vi "Dashboard Main.vi"() -> ()   [LabVIEW 2015]
uses:
  <vilib>/Utility/miscctls.llb/LVRowAndColumnTypeDef.ctl
  <vilib>/event_ctls.llb/eventvkey.ctl
  <vilib>/Rock Robotics/WPI/Dashboard/WPI_DashboardLogging Global.vi
  <vilib>/Rock Robotics/Network Tables/NT Read Numeric Array.vi
  <vilib>/Utility/config.llb/Write Key (String).vi
  <vilib>/Utility/config.llb/Write Key (I32).vi
  <vilib>/Utility/config.llb/NI_LVConfig.lvlib
panel:
  out "Robot IP":string
  in  "stop":bool
  in  "TCP":refnum<k5>
  out "Camera IP":string
  out "Image Message":string="Timeout in Camera Communications"
  in  "Dashboard Tab":T1(tab)
  in  "Select Auto":string(combo)
  out "NT Connection":bool
  in  "Camera Settings":T2={"Frame Rate"=30, "Compression"=30, "Size"=1} {"Frame Rate" scale=1.0..30.0; "Size" items=["640x480", "320x240", "160x120"]}
  out "MotorChart R":cluster{"Numeric":dbl, "Numeric":dbl}(graph)
  out "MotorChart L":T3(graph)
  out "MotorSliders R":cluster{"MotorSlide1":dbl, "MotorSlide2":dbl} {"MotorSlide2" scale=-1.0..1.0 scale format="%#_2e"; "MotorSlide1" scale=-1.0..1.0 scale format="%#_2e"}
  out "MotorSliders L":T4 {"MotorSlide4 2" scale=0.0..14.0 scale format="%#_2e"; "MotorSlide2" scale=-1.0..1.0 scale format="%#_2e"; "MotorSlide1" scale=-1.0..1.0 scale format="%#_2e"}
  out "Gyro":dbl(knob) scale=0.0..360.0
  out "JS1 Z":dbl(slide) scale=-1.0..1.0 scale format="%#_2e"
  out "JS1 Graph":cluster{"X":dbl, "Y":dbl}[](graph)
  out "JS1 Buttons":T5
  out "JS2 Z":dbl(slide) scale=-1.0..1.0 scale format="%#_2e"
  out "JS2 Graph":cluster{"X":dbl, "Y":dbl}[](graph)
  out "JS2 Buttons":T5
  out "Mode":T6(ring)=enum."Auto Disabled"
  in  "DB Camera Config":bool
  out "fps":dbl format="%#.1g"
  out "Mbps":dbl format="%#.1g"
  out "Mbps LED":bool
  in  "Vision":u16(ring) items=["Camera Off", "USB Camera SW", "USB Camera HW", "IP Camera"]
  in  "Rec Mode":enum32{"Stop", "Record", "Playback"}(radio)
  out "Camera Image":T7(plugin-control)
  out "Background":bool
  in  "DB/String 9":string
  in  "DB/String 8":string
  in  "DB/String 7":string
  in  "DB/String 6":string
  in  "DB/String 5":string
  in  "DB/String 4":string
  in  "DB/String 3":string
  in  "DB/String 2":string
  in  "DB/String 1":string
  in  "DB/String 0":string
  in  "DB/Slider 0":dbl(slide) scale=0.0..5.0
  in  "DB/Slider 1":dbl(slide) scale=0.0..5.0
  in  "DB/Slider 2":dbl(slide) scale=0.0..5.0
  in  "DB/Slider 3":dbl(slide) scale=0.0..5.0
  out "DB/LED 3":bool
  out "DB/LED 2":bool
  out "DB/LED 1":bool
  out "DB/LED 0":bool
  in  "DB/Button 3":bool
  in  "DB/Button 2":bool
  in  "DB/Button 1":bool
  in  "DB/Button 0":bool caption="New Name"
  in  "Test Slider":dbl(slide) scale=0.0..100.0 scale format="%#_3g"
  in  "On/Off":bool caption="Solenoid"
  in  "Test Name":u16(ring) items=["Select the test to run..."]
  in  "Test Tree":string(tree)
  in  "Motor":cluster{"Value":dbl, "Enable":bool} {"Value" scale=-1.0..1.0 scale format="%#_3g"}
  out "Progress":T8 {"Test Progress" scale=0.0..100.0}
  in  "Rev/Fwd":cluster{"Forward":bool, "Reverse":bool}
  in  "Test Ring":u16(ring) items=["Monochrome", "Color"]
  out "Cmd Status":string
  in  "Execute Command":bool
  in  "Command Params":string[][](table)
  in  "Command Selection":i32(listbox)
  in  "CheckList":i32(listbox)
  out "Tree":string(tree)
  out "Sorted Particle Scores":T9(array[cluster]) {"Moment Factor" format="%#_3g"; "Aspect Ratio" format="%#_3g"; "Area to CH" format="%#_3g"; "X" format="%#_3g"; "Y" format="%#_3g"}
  out "Detected Targets":T10(array[cluster]) {"Normalized Rect"."Numeric 5" format="%#_2g"; "Normalized Rect"."Numeric 3" format="%#_2g"; "Normalized Rect"."Numeric 2" format="%#_2g"; "Normalized Rect"."Numeric" format="%#_2g"}
  in  "LED Color":T11={"Hue"={101.77223077407461, 133.17163207204948}, "Sat"={151.78571428571428, 255.0}, "Val"={48.571428571428584, 255.0}} {"Hue" scale=0.0..255.0 scale format="%#_3g"}
  out "Masked":T7(plugin-control)
  in  "Viewing Angle":dbl
  # "Left"
  # "Front"
  # "Right"
  # "Battery"
  # "This tab is a great place for autonomous settings and robot-specific values.\nPlace controls and indicators inside this tab and match name to\nDashboard Variables on robot. You can also delete this comment."
  # "Density Profile"
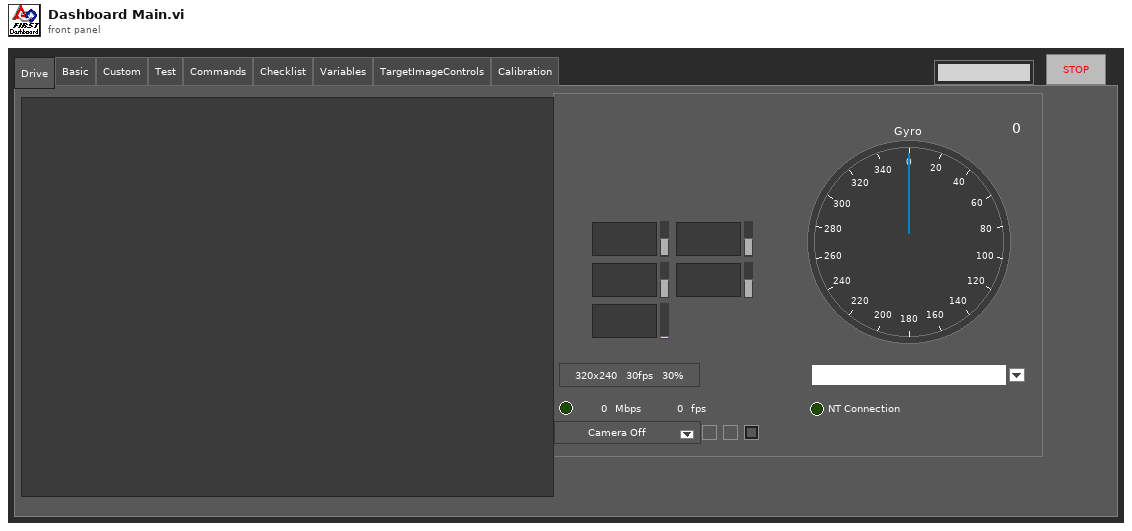
[diagram p1: front panel]
types:
  T1 = enum32{"Drive", "Basic", "Custom", "Test", "Commands", "Checklist", "Variables", "TargetImageControls", "Calibration"}
  T2 = cluster{"Frame Rate":i32, "Compression":i32, "Size":u16}
  T3 = cluster{"Numeric":dbl, "Numeric":dbl, "Battery V":dbl}
  T4 = cluster{"MotorSlide1":dbl, "MotorSlide2":dbl, "MotorSlide4 2":dbl}
  T5 = cluster{bool, bool, bool, bool, bool, bool, bool, bool, bool, bool, bool, bool}
  T6 = enum8{"Tele-Op Disabled", "Tele-Op Enabled", "Auto Disabled", "Auto Enabled", "Test Disabled", "Test Enabled", "Disconnected", "No Code", "E-Stop"}
  T7 = typedef "IMAQ Image.ctl" = refnum<image>
  T8 = cluster{"Test Progress":u8, "Test Progress Text":string}
  T9 = cluster{"Rectangle px":cluster{"Numeric":dbl, "Numeric 2":dbl, "Numeric 3":dbl, "Numeric 5":dbl}, "Aspect Ratio":dbl, "Area to CH":dbl, "X":dbl, "Y":dbl, "Moment Factor":dbl}[]
  T10 = cluster{"Distance (ft)":dbl, "Center":cluster{dbl, dbl}, "Normalized Rect":cluster{"Numeric":dbl, "Numeric 2":dbl, "Numeric 3":dbl, "Numeric 5":dbl}}[]
  T11 = cluster{"Hue":cluster{dbl, dbl}, "Sat":cluster{dbl, dbl}, "Val":cluster{dbl, dbl}}
  T12 = cluster{"IDs":cluster{"RPC field ID":u16, "Unique ID":u16}, "String":string}
  T13 = enum32{"Drive", "Basic", "Custom", "Test", "Commands", "Checklist", "Variables"}
  T14 = enum32{"Drive", "Basic", "Custom", "Test", "Checklist", "Variables"}
  T15 = typedef "Image Type" = u32
  T16 = cluster{"Camera Image":refnum<vi>, "Dashboard Tab":refnum<vi>, "Background":refnum<vi>, "Vision":refnum<vi>, "Rec Mode":refnum<vi>, "Test Slider":refnum<vi>, "On/Off ":refnum<vi>, "Test Ring":refnum<vi>, "Rev/Fwd":refnum<vi>, "Test Name":refnum<vi>, "Motor":refnum<vi>, "Progress":refnum<vi>, "CheckList":refnum<vi>, "Tree":refnum<vi>, "Test Tree":refnum<vi>, "Command Params":refnum<vi>, "Command Selection":refnum<vi>, "Execute Command":refnum<vi>, "Cmd Status":refnum<vi>}
  T17 = cluster{"Error Strings":string, "Disable Counts":cluster{u16, u16}, "Rail Faults":cluster{u16, u16, u16}, "Robot IP":string, "DB Mode":u8, "Event Info":cluster{"Name":string, "Type":u8, "Number":u16, "Replay":u8}, "Camera Addr":string}
  T18 = cluster{"Storage":cluster{"Disk Free":u64, "RAM Block":u32, "RAM free":u32}, "CPU Utilization":cluster{"CPU % ISR":sgl, "CPU % Time Crit":sgl, "CPU % Timed Str":sgl, "CPU % High":sgl, "CPU % Above":sgl, "CPU % Normal":sgl, "CPU % Low":sgl}, "CAN":cluster{"% Bus Utilization":sgl, "Bus Off Cnt":u32, "TX_FIFO Full Cnt":u32, "Receive Error Cnt":u8, "Transmit Error Cnt":u8}, "HID":cluster{"HID Outputs":u32, "Rumble Low":u16, "Rumble High":u16}[]}
  T19 = cluster{"Status bits":cluster{"Test Mode":bool, "Autonomous":bool, "Enabled":bool, "Code Start":bool, "Brownout":bool, "Reserved 2":bool, "Reserved 3":bool, "E-Stop":bool}, "Code Trace":cluster{"Disabled":bool, "TeleOp":bool, "Auto":bool, "Test":bool}, "Controller Type":enum16{"unknown", "cRIO", "roboRio"}, "Code?":enum16{"unknown", "noCode", "code"}, "Battery V":dbl}
  T20 = cluster{"Control Bits":cluster{"TestMode":bool, "Autonomous":bool, "Enabled":bool, "FMS Present":bool, bool, bool, bool, "E-Stop":bool}, "Team Station ":u8, "Countdown":sgl, "Joystick Values":cluster{"Axes":dbl[], "Buttons":bool[], "POVs":i16[]}[]}
  T21 = cluster{"Axes":dbl[], "Buttons":bool[], "POVs":i16[]}[]
  T22 = cluster{"Axes":dbl[], "Buttons":bool[], "POVs":i16[]}
  T23 = cluster{"Buttons[0]":bool, "Buttons[1]":bool, "Buttons[2]":bool, "Buttons[3]":bool, "Buttons[4]":bool, "Buttons[5]":bool, "Buttons[6]":bool, "Buttons[7]":bool, "Buttons[8]":bool, "Buttons[9]":bool, "Buttons[10]":bool, "Buttons[11]":bool}
  T24 = typedef "NI_LVConfig.lvlib/Config Data RefNum.ctl" = refnum<k1>
  T25 = cluster{"Operation":enum16{"Update", "Clear"}, "Color Box":u32}[]
  T26 = typedef "eventvkey.ctl" = enum16{"ASCII", "Enter", "Return", "Shift", "Ctrl", "Alt", "Cmd", "Opt", "Caps", "NumLock", "Clear", "Break", "Up", "Down", "Left", "Right", "Insert", "Delete", "Home", "End", "PageUp", "PageDown", "Escape", "Help", "Pause", "ScrollLock", "F1", "F2", "F3", "F4", "F5", "F6", "F7", "F8", "F9", "F10", "F11", "F12", "F13", "F14", "F15", "F16", "F17", "F18", "F19", "F20", "F21", "F22", "F23", "F24", "Play", "VolumeUp", "VolumeDown", "Mute", "Two Byte Char"}
  T27 = cluster{"Image Size":bool, "Image Type":bool, "Pixel Value":bool, "ROI Information":bool, "Zoom Factor":bool}
  T28 = enum8{"Enabled", "Disabled", "Disabled and Grayed Out"}
  T29 = cluster{"Operation":enum16{"Update", "Clear"}, "Color Box":u32}
  T30 = typedef "LVRowAndColumnTypeDef.ctl" = cluster{"Row":i32, "Column":i32}
  T31 = cluster{"Shift":bool, "Ctrl":bool, "Alt":bool, "Cmd":bool, "Opt":bool}
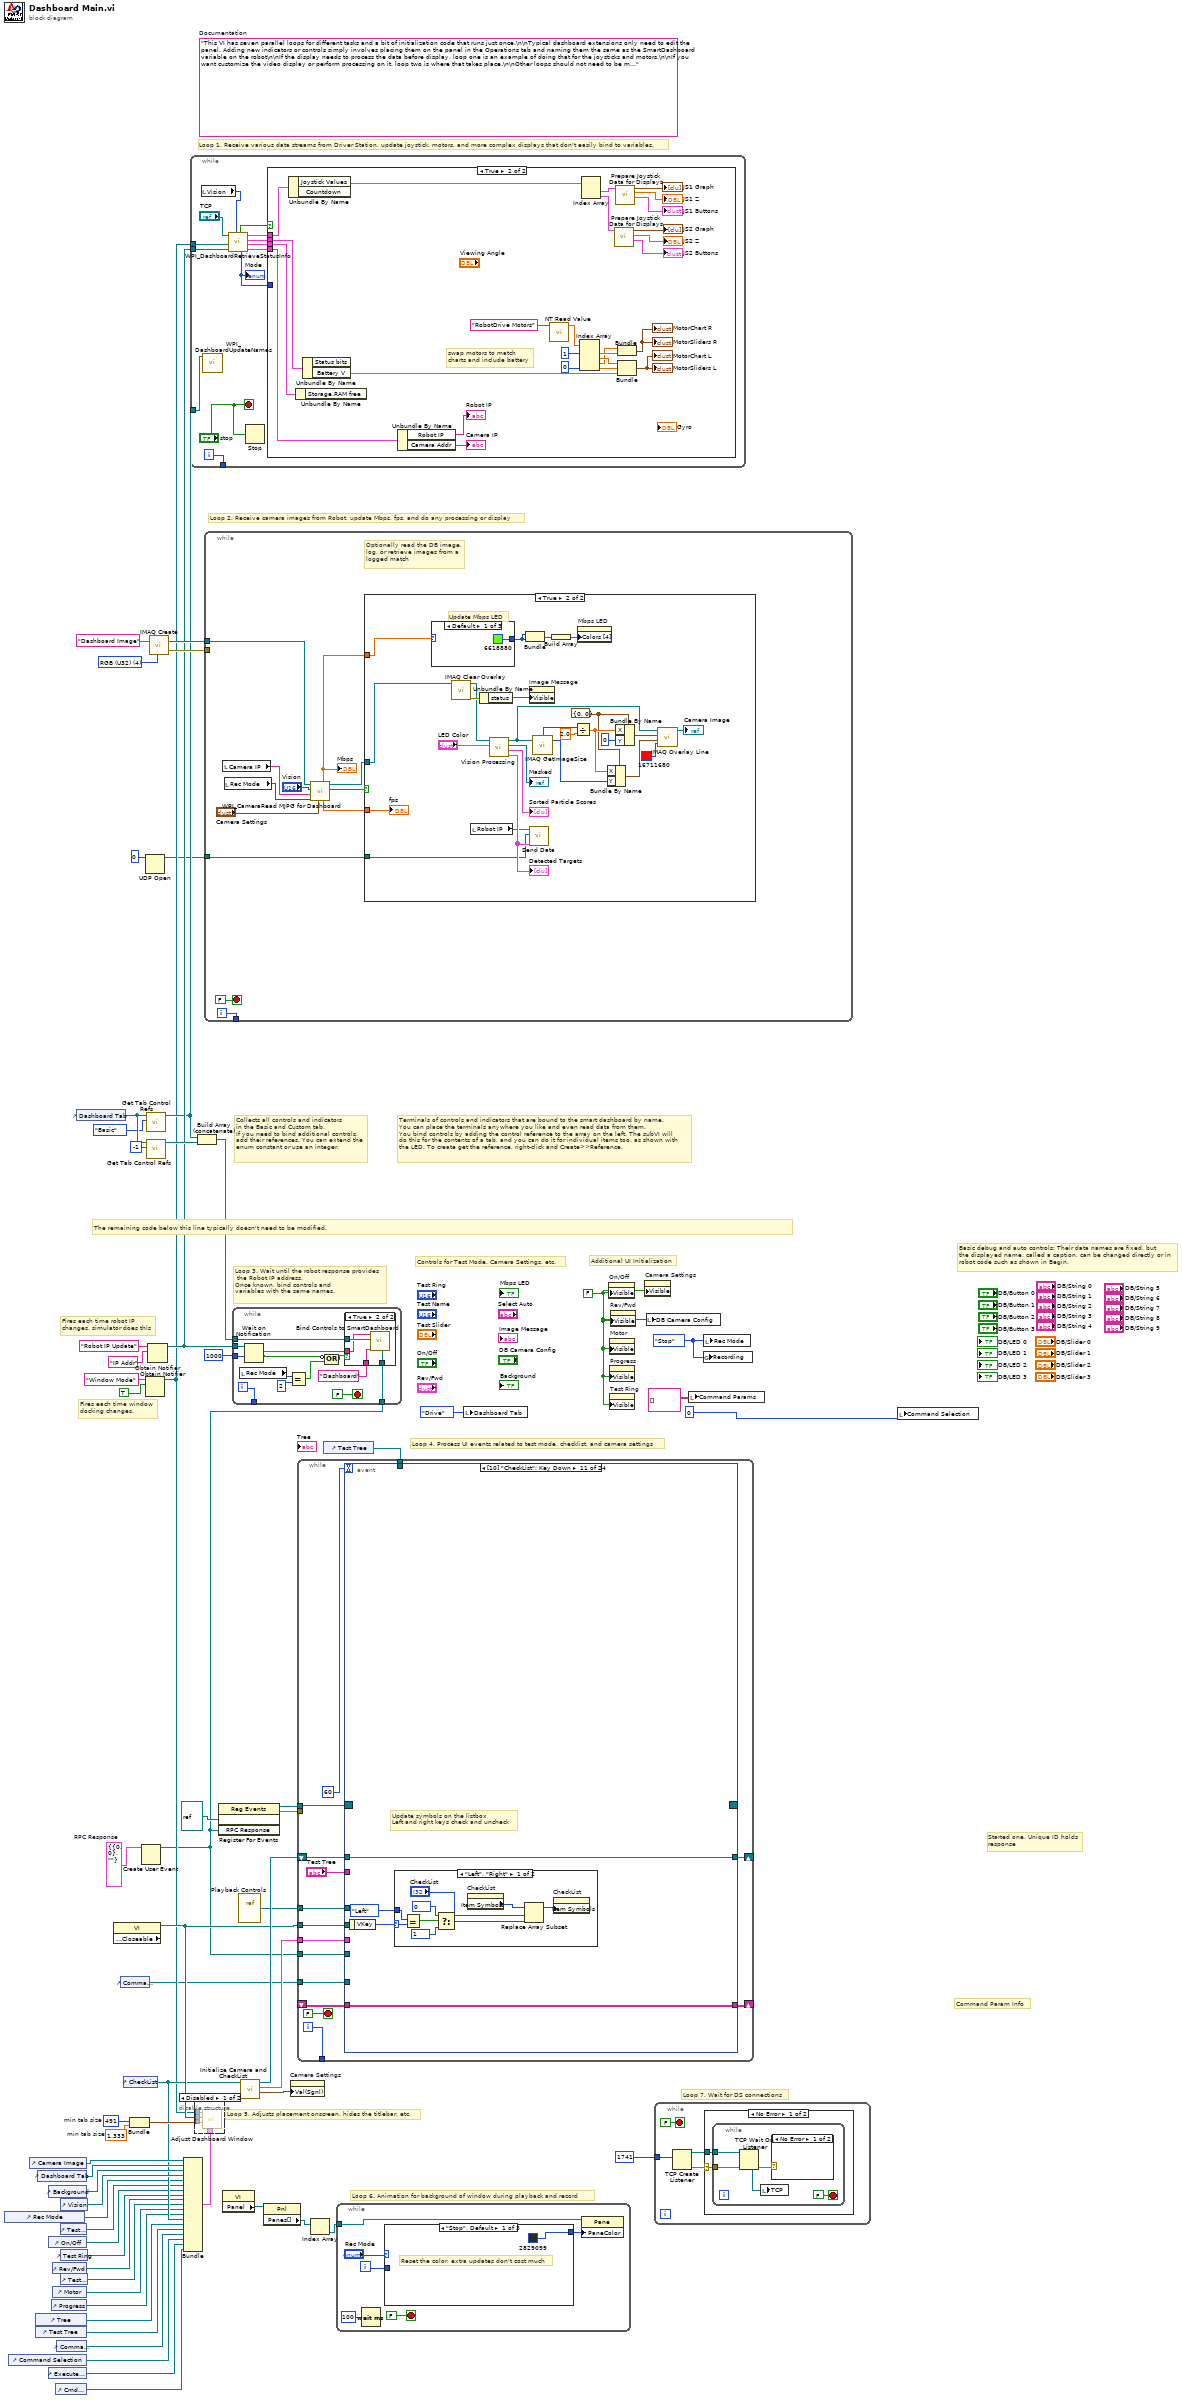
[diagram p0: block diagram]
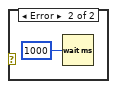
[diagram p3: hidden frame]
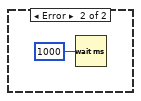
[diagram p4: hidden frame]
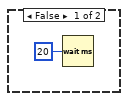
[diagram p5: hidden frame]
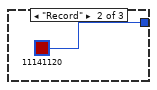
[diagram p6: hidden frame]
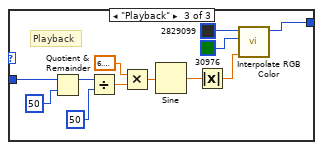
[diagram p7: hidden frame]
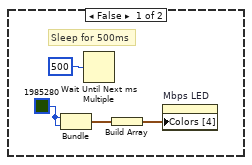
[diagram p9: hidden frame]
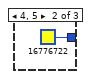
[diagram p10: hidden frame]
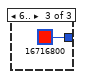
[diagram p11: hidden frame]
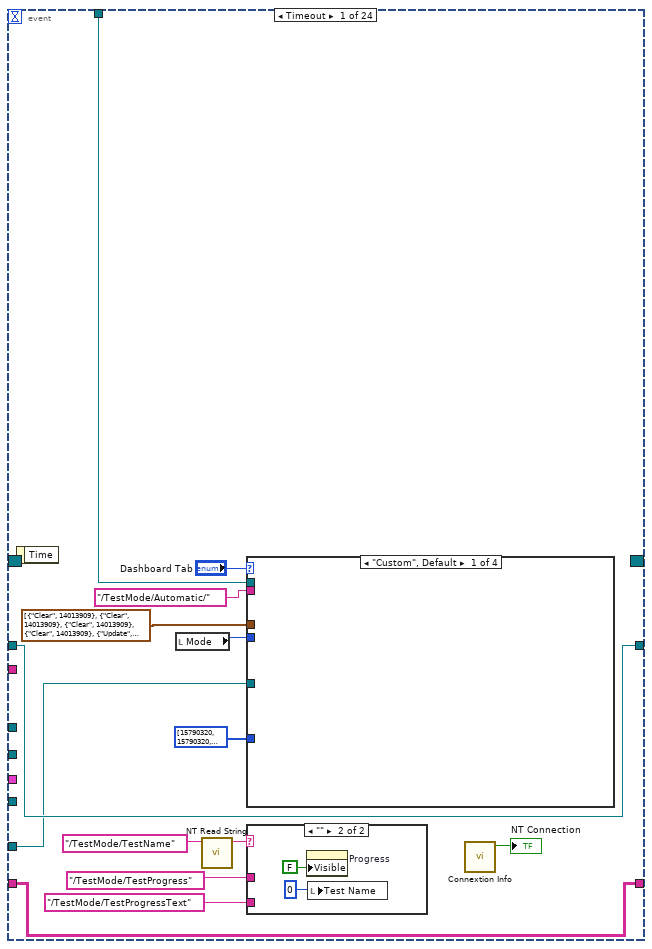
[diagram p12: hidden frame]
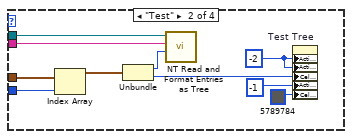
[diagram p13: hidden frame]
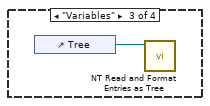
[diagram p14: hidden frame]
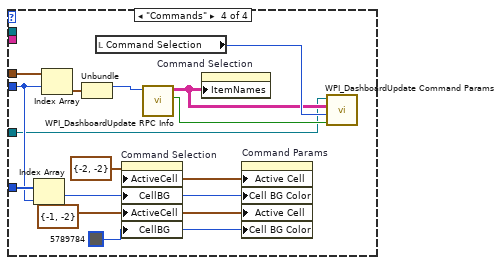
[diagram p15: hidden frame]
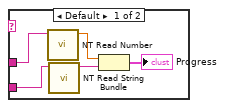
[diagram p16: hidden frame]
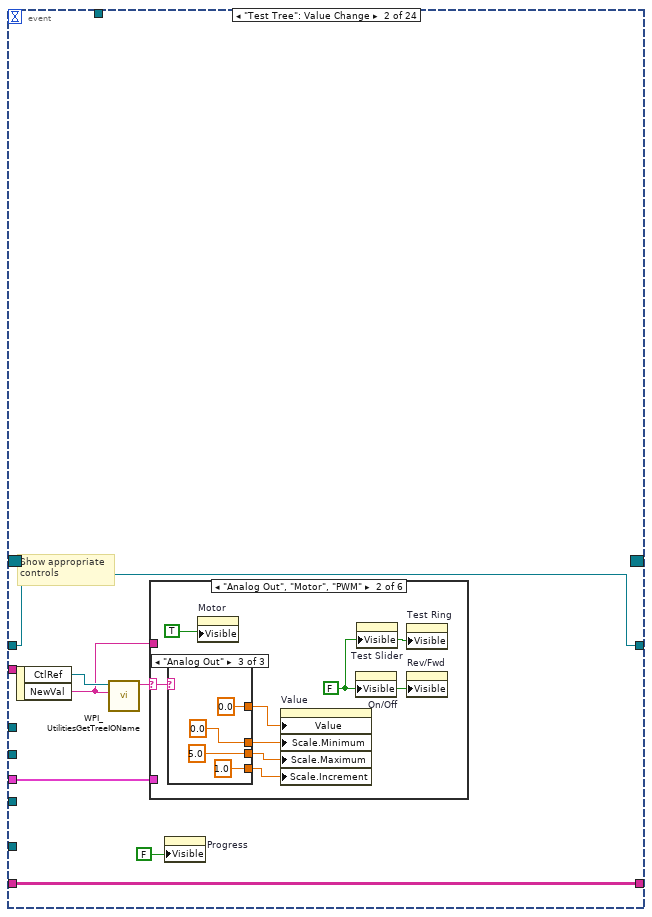
[diagram p17: hidden frame]
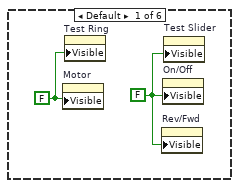
[diagram p18: hidden frame]
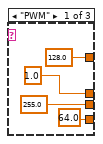
[diagram p19: hidden frame]
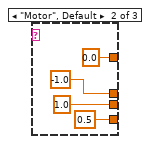
[diagram p20: hidden frame]
diagram:
  w9 = T12 {"IDs"={"RPC field ID"=0, "Unique ID"=0}, "String"=""}  # RPC Response
  w35 = 491  # min tab size
  w34 = 1.333  # min tab size
  w43 = enum32{"Stop", "Record", "Playback"}."Stop" ("Rec Mode")
  w17 = FALSE ("Visible")
  (unwired) "This VI has seven parallel loops for different tasks and a bit of initialization code that runs just once.\n\nTypical dashboard extensions only need to edit the panel. Adding new indicators or controls simply involves placing them on the panel in the Operations tab and naming them the same as the SmartDashboard variable on the robot\n\nIf the display needs to process the data before display, loop one is an example of doing that for the joysticks and motors.\n\nIf you want customize the video display or perform processing on it, loop two is where that takes place.\n\nOther loops should not need to be modified. They are pretty standard, and document the task they perform."  # Documentation
  w63 = T15 4 items=["Grayscale (U8)", "Grayscale (I16)", "Grayscale (SGL)", "Complex (CSG)", "RGB (U32)", "HSL (U32)", "RGB (U64)"] ("Image Type")
  # "Command Param Info"
  # "Started one, Unique ID holds\nresponse"
  # "Loop 7. Wait for DS connections"
  # "Basic debug and auto controls: Their data names are fixed, but\nthe displayed name, called a caption, can be changed directly or in\nrobot code such as shown in Begin."
  # "Controls for Test Mode, Camera Settings, etc."
  # "Additional UI Initialization"
  # "Loop 6. Animation for background of window during playback and record"
  # "Fires each time robot IP\nchanges, simulator does this"
  # "Fires each time window\ndocking changes."
  # "Collects all controls and indicators\nin the Basic and Custom tab.\nIf you need to bind additional controls,\nadd their references. You can extend the\nenum constant or use an integer."
  # "The remaining code below this line typically doesn't need to be modified."
  # "Loop 4. Process UI events related to test mode, checklist, and camera settings"
  # "Terminals of controls and indicators that are bound to the smart dashboard by name.\nYou can place the terminals anywhere you like and even read data from them.\nYou bind controls by adding the control reference to the array on the left. The subVI will\ndo this for the contents of a tab, and you can do it for individual items too, as shown with\nthe LED. To create get the reference, right-click and Create>>Reference."
  # "Loop 3. Wait until the robot response provides\n the Robot IP address.\nOnce known, bind controls and\nvariables with the same names."
  # "Loop 5. Adjusts placement onscreen, hides the titlebar, etc."
  # "Loop 1. Receive various data streams from Driver Station, update joystick, motors, and more complex displays that don't easily bind to variables."
  # "Loop 2. Receive camera images from Robot, update Mbps, fps, and do any processing or display"
  n1 = control-ref of="Rec Mode"() -> (w23:refnum<vi>)
  n2 = control-ref of="Command Selection"() -> (w8:refnum<vi>)
  n3 = control-ref of="Camera Image"() -> (w38:refnum<vi>)
  n4 = control-ref of="Tree"() -> (w27:refnum<vi>)
  n5 = control-ref of="Test Tree"() -> (w26:refnum<vi>)
  n6 = control-ref of="Dashboard Tab"() -> (w37:refnum<vi>)
  n7 = control-ref of="Execute Command"() -> (w10:refnum<vi>)
  n8 = control-ref of="Background"() -> (w32:refnum<vi>)
  n9 = control-ref of="On/Off"() -> (w21:refnum<vi>)
  n10 = control-ref of="Progress"() -> (w18:refnum<vi>)
  n11 = control-ref of="Rev/Fwd"() -> (w19:refnum<vi>)
  n12 = control-ref of="Motor"() -> (w24:refnum<vi>)
  n13 = control-ref of="Cmd Status"() -> (w4:refnum<vi>)
  n14 = control-ref of="Command Params"() -> (w11:refnum<vi>)
  n15 = control-ref of="Test Slider"() -> (w22:refnum<vi>)
  n16 = control-ref of="Vision"() -> (w36:refnum<vi>)
  n17 = control-ref of="Test Ring"() -> (w20:refnum<vi>)
  n18 = control-ref of="Test Name"() -> (w25:refnum<vi>)
  n19 = control-ref of="Dashboard Tab"() -> (w41:refnum<vi>)
  n20 = property class="VI" props=["Front Panel.Closeable"]() -> (reference out=w42:refnum<vi>)  [unwired: 2 in, 2 out]
  n21 = control-ref of="Command Params"() -> (w3:refnum<vi>)
  n22 = control-ref of="CheckList"() -> (w28:refnum<vi>)
  n23 = Bundle("min tab size"=w35, "min tab size"=w34) -> (w33:cluster{"min tab size":i32, "min tab size":dbl})  [unwired: 1 in]
  n24 = Create User Event(user event datatype=w9) -> (user event=w5:refnum<user-event>)  [unwired: 1 in, 1 out]
  n25 = UDP Open(11:u16 0 ("port")) -> (port=w1:refnum<k16>)  [unwired: 4 in, 2 out]
  n26 = Obtain Notifier(name (unnamed)="Window Mode", notification data type=TRUE) -> (notifier out=w14:refnum<notifier>)  [unwired: 2 in, 2 out]
  n27 = call <vilib>:"Get Tab Control Refs.vi"("Page Index"=T14."Basic" ("Dashboard Tab"), "TabControl in"=w41) -> ("ControlsOnPage"=w15:refnum<vi>[])  [unwired: 9 in]
  n28 = call <vilib>:"Get Tab Control Refs.vi"("Page Index"=-1, "TabControl in"=w41) -> ("ControlsOnPage"=w40:refnum<vi>[])  [unwired: 9 in]
  n29 = Obtain Notifier(name (unnamed)="Robot IP Update", notification data type="IP Addr" ("name (unnamed)")) -> (notifier out=w16:refnum<notifier>)  [unwired: 2 in, 2 out]
  n30 = call "IMAQ Create"("Image Name"="Dashboard Image", "Image Type"=w63) -> ("New Image"=w61:T7, "error out"=w60:errorcluster)  [unwired: 2 in, 1 out]
  n31 = Bundle("Camera Image"=w38, "Dashboard Tab"=w37, "Background"=w32, "Vision"=w36, "Rec Mode"=w23, "Test Slider"=w22, "On/Off"=w21, "Test Ring"=w20, "Rev/Fwd"=w19, "Test Name"=w25, "Motor"=w24, "Progress"=w18, "CheckList"=w28, "Tree"=w27, "Test Tree"=w26, "Command Params"=w11, "Command Selection"=w8, "Execute Command"=w10, "Cmd Status"=w4) -> (w29:T16)  [unwired: 1 in]
  n32 = while {
    tunnel: [w76] -> _
    tunnel: w16 -> [w70]
    tunnel: w15 -> [w69]
    tunnel: w14 -> [w65]
    i -> [w76]
    stop <- "stop" stop-if-true
    n33 = local read "Vision"() -> (w67:u16)
    n34 = call <vilib>:"WPI_DashboardUpdateNames.vi"("Controls on Tab"=w69) -> ()  [unwired: 11 in]
    n35 = call <vilib>:"WPI_DashboardRetrieveStatusInfo.vi"("Vision"=w67, "Binding Refnum"=w70, "Window Mode Notifier"=w65, "TCP Cnx"="TCP") -> ("Power and Errors"=w71:T17, "Robot Metrics"=w74:T18, "Status Info"=w75:T19, "Control Info"=w72:T20, "Robot Mode"=w68:T6, "Process?"=w73:bool)  [unwired: 2 in]
    "Mode" <- w68
    n36 = Stop(stop? (T)="stop") -> ()
    n37 = case shown="True" w73 {
      tunnel: w75 -> [_ w103]
      tunnel: w74 -> [_ w102]
      tunnel: w72 -> [_ w101]
      tunnel: w71 -> [_ w100]
      tunnel: w68 -> [_ _]
      frame False {
        n38 = Wait (ms)(milliseconds to wait=u32 20) -> ()  [unwired: 1 out]
      }
      frame True {
        # "swap motors to match\ncharts and include battery"
        n39 = Unbundle By Name(w101) -> ("Joystick Values"=w90:T21)  [unwired: 1 out]
        n40 = Unbundle By Name(w102) -> ()  [unwired: 1 out]
        n41 = Unbundle By Name(w103) -> ("Battery V"=w91:dbl)  [unwired: 1 out]
        n42 = Unbundle By Name(w100) -> ("Robot IP"=→"Robot IP":string, "Camera Addr"=→"Camera IP":string)
        n43 = call-poly <vilib>:"NT Read Value.vi"("Name"="RobotDrive Motors") -> ("Numeric Array"=w79:dbl[])  [unwired: 9 in, 1 out]
        n44 = Index Array(array=w79, index #1=1, index #4=0) -> (element #1=w95:dbl, element #2=w96:dbl, element #3=w94:dbl, element #4=w99:dbl)  [unwired: 2 in]
        n45 = Index Array(array=w90) -> (element #1=w89:T22, element #2=w84:T22)  [unwired: 2 in]
        n46 = call "Prepare Joystick Data for Displays.vi"("Joystick Values"=w84) -> ("Buttons"=→"JS2 Buttons":T23, "Z Axis"=→"JS2 Z":dbl, "Cartesian Data"=→"JS2 Graph":cluster{"X axis":dbl, "X axis":dbl}[])  [unwired: 8 in]
        n47 = call "Prepare Joystick Data for Displays.vi"("Joystick Values"=w89) -> ("Buttons"=→"JS1 Buttons":T23, "Z Axis"=→"JS1 Z":dbl, "Cartesian Data"=→"JS1 Graph":cluster{"X axis":dbl, "X axis":dbl}[])  [unwired: 8 in]
        n48 = Bundle("Numeric"=w94, "Numeric"=w95) -> (→"MotorChart R" →"MotorSliders R":cluster{"Numeric":dbl, "Numeric":dbl})  [unwired: 1 in]
        n49 = Bundle("Numeric"=w96, "Numeric"=w99, "Battery V"=w91) -> (→"MotorChart L" →"MotorSliders L":T3)  [unwired: 1 in]
      }
    }
  }
  n50 = disable-structure shown="Disabled" {
    disable-tunnel: w42 -> [w107 _]
    disable-tunnel: w33 -> [w106 _]
    disable-tunnel: w29 -> [w105 _]
    disable-tunnel: w14 -> [w104 _]
    frame Disabled {
      n51 = call "Adjust Dashboard Window.vi"("Sizing Refnums"=w105, "Size Constraints"=w106, "VI"=w107, "WIn Mode"=w104) -> ()  [unwired: 8 in]
    }
    frame Enabled {
    }
  }
  n52 = Build Array (concatenate)(w15, w40) -> (w39:refnum<vi>[])
  n53 = while {
    tunnel: w61 -> [w117]
    tunnel: w60 -> [_]
    tunnel: [w118] -> _
    tunnel: w1 -> [w108]
    i -> [w118]
    stop <- FALSE stop-if-true
    # "Optionally read the DB image,\nlog, or retrieve images from a\nlogged match"
    n54 = local read "Camera IP"() -> (w110:string)
    n55 = local read "Rec Mode"() -> (w112:enum32{"Stop", "Record", "Playback"})
    n56 = call <vilib>:"WPI_CameraRead MJPG for Dashboard.vi"("Camera Settings"="Camera Settings", "Rec Mode"=w112, "Camera IP"=w110, "Camera Mode"="Vision", "Refnum in"=w117) -> ("Active"=w115:bool, "Refnum out"=w116:T7, "FPS"=w114:dbl, "Bandwidth (Mbps)"=w109:dbl)  [unwired: 3 in]
    "Mbps" <- w109
    n57 = case shown="True" w115 {
      tunnel: w116 -> [_ w144]
      tunnel: w109 -> [_ w143]
      tunnel: w114 -> [_ w142]
      tunnel: w108 -> [_ w125]
      frame False {
        w120 = u32 1985280 ("Color Box")
        # "Sleep for 500ms"
        n58 = Bundle("Color Box"=w120, "Color Box"=w120) -> (w122:cluster{"Color Box":u32, "Color Box":u32})  [unwired: 1 out]
        n59 = Wait Until Next ms Multiple(millisecond multiple=u32 500) -> ()  [unwired: 1 out]
        n60 = Build Array(w122) -> (w121:cluster{"Color Box":u32, "Color Box":u32}[])
        n61 = property on="Mbps LED" class="Bool (strict)"("Colors [4]"=w121) -> ()  [unwired: 2 in, 2 out]
      }
      frame True {
        w127 = cluster{"X":i32, "Y":i32} {"X"=0, "Y"=0} ("Start Point")
        # "Update Mbps LED"
        n62 = case shown="Default" w143 {
          tunnel: [u32 6618880 ("Color Box") u32 16776722 ("Color Box") u32 16716800 ("Color Box")] -> w145
          frame Default {
          }
          frame 4, 5 {
          }
          frame 6.. {
          }
        }
        n63 = call "IMAQ Clear Overlay"("Image"=w144) -> ("error out"=w148:errorcluster, "Image Out"=w141:T7)  [unwired: 2 in, 7 out]
        n64 = local read "Robot IP"() -> (w137:string)
        n65 = Unbundle By Name(w148) -> ("status"=w149:bool)
        n66 = call "Vision Processing.vi"("LED Color"="LED Color", "Image Src"=w141) -> ("Detected Targets"=w138:T10, "Sorted Particle Scores"=→"Sorted Particle Scores":T9, "Masked"=→"Masked":T7, "Original Image"=w135:T7)  [unwired: 2 in]
        "Detected Targets" <- w138
        n67 = Bundle("Color Box"=w145, "Color Box"=w145) -> (w147:cluster{"Color Box":u32, "Color Box":u32})  [unwired: 1 out]
        n68 = property on="Image Message" class="Str"("Visible"=w149) -> ()  [unwired: 2 in, 2 out]
        n69 = call "Send Data.vi"("Detected Targets"=w138, "connection ID"=w125, "name"=w137) -> ()  [unwired: 9 in]
        n70 = call "IMAQ GetImageSize"("Image"=w135) -> ("Y Resolution"=w130:i32, "X Resolution"=w133:i32)  [unwired: 3 in, 1 out]
        n71 = Build Array(w147) -> (w146:cluster{"Color Box":u32, "Color Box":u32}[])
        n72 = Divide(x=w133, y=2.0) -> (x/y=w129:dbl)
        n73 = property on="Mbps LED" class="Bool (strict)"("Colors [4]"=w146) -> ()  [unwired: 2 in, 2 out]
        n74 = Bundle By Name(cluster=w127, "X"=w129, "Y"=w130) -> (w128:cluster{"X":i32, "Y":i32})
        n75 = Bundle By Name(cluster=w127, "X"=w129, "Y"=0) -> (w131:cluster{"X":i32, "Y":i32})
        n76 = call "IMAQ Overlay Line"("Color"=u32 16711680, "End Point"=w128, "Start Point"=w131, "Image"=w135) -> ("Image Out"=→"Camera Image":T7)  [unwired: 6 in, 1 out]
        "fps" <- w142
      }
    }
  }
  n77 = register-events(refnum<vi> refnum, w5) -> (reference out=w47:refnum<event-registration>, error out=w46:errorcluster)  [unwired: 2 in]
  n78 = property class="VI"() -> ("Panel"=w50:refnum<vi>)  [unwired: 2 in, 2 out]
  n79 = while {
    tunnel: w39 -> [w165]
    tunnel: w16 -> [w163]
    tunnel: [w161] -> _
    tunnel: u32 1000 ("milliseconds to wait") -> [w160]
    tunnel: w5 -> [w153]
    i -> [w161]
    stop <- FALSE stop-if-true
    n80 = local read "Rec Mode"() -> (w156:enum32{"Stop", "Record", "Playback"})
    n81 = Wait on Notification(notifier=w163, timeout in ms (-1)=w160) -> (notification=w162:string, timed out?=w158:bool)  [unwired: 2 in, 2 out]
    n82 = Equal?(x=w156, y=u16 2 ("Rec Mode")) -> (x = y?=w157:bool)
    n83 = Compound Arithmetic op=OR(invert w158, w157) -> (w159:bool)
    n84 = case shown="True" w159 {
      tunnel: w165 -> [_ w169]
      tunnel: w162 -> [_ w168]
      tunnel: "Dashboard" -> [_ w167]
      tunnel: w153 -> [_ w166]
      frame False {
      }
      frame True {
        n85 = call <vilib>:"Bind Controls to SmartDashboard.vi"("RPC ref"=w166, "Client Name"=w167, "Bound Control Refs"=w169, "Server IP Address"=w168) -> ()  [unwired: 8 in]
      }
    }
  }
  n86 = vi-ref "Playback Controls.vi"() -> (w48:refnum<vi>)
  n87 = call "Initialize Camera and CheckList.vi"("ListBox in"=w28) -> ("Cluster"=w54:cluster{"value":i32, "value":i32, "index":i32}, "Array"=w55:cluster{string[]}[], "File Refnum"=w53:T24)  [unwired: 8 in]
  n88 = property class="Pnl"(reference=w50) -> ("Panes[]"=w51:refnum<vi>[])  [unwired: 1 in, 2 out]
  n89 = property on="Camera Settings" class="Clust (strict)"("Val(Sgnl)"=w54) -> ()  [unwired: 2 in, 2 out]
  n90 = Index Array(array=w51) -> (element=w49:refnum<vi>)  [unwired: 1 in]
  n91 = control-ref of="Test Tree"() -> (w52:refnum<vi>)
  n92 = while {
    tunnel: w55 -> [w181]
    shift-right: [w180] -> _
    shift-left: w53 -> [w179]
    tunnel: [w178] -> _
    tunnel: w52 -> [w177]
    tunnel: w48 -> [w176]
    tunnel: w47 -> [w175]
    tunnel: w46 -> [_]
    tunnel: w42 -> [w174]
    tunnel: w5 -> [w173]
    tunnel: w3 -> [w172]
    shift-right: [w171] -> _
    shift-left: _ -> [w170]
    i -> [w178]
    stop <- FALSE stop-if-true
    n93 = event shown="[10] \"CheckList\": Key Down" {
      selector: w175 -> [_ _ _ _ _ _ _ _ _ _ _ _ _ _ _ _ _ _ _ _ _ _ _ _]
      dyn-events: [_ _ _ _ _ _ _ _ _ _ _ _ _ _ _ _ _ _ w490 _ _ _ _ _] -> _
      timeout: u32 60 ("milliseconds to wait") -> [_ _ _ _ _ _ _ _ _ _ _ _ _ _ _ _ _ _ _ _ _ _ _ _]
      tunnel: w177 -> [w194 _ _ _ _ _ _ _ _ _ _ _ _ _ _ _ _ _ _ _ _ _ _ _]
      tunnel: "Test Tree" -> [_ _ _ _ _ _ _ _ _ _ _ _ _ w453 w462 w465 w470 w479 _ _ _ _ _ _]
      tunnel: w181 -> [_ w232 _ _ _ _ _ _ _ _ _ w415 w446 _ _ _ _ _ _ _ _ _ _ _]
      tunnel: [w191 w231 w335 w341 w351 w355 w361 w373 w381 w387 w400 w414 w439 w452 w460 w464 w469 w478 w492 w508 w510 w518 w529 w534] -> w180
      tunnel: w179 -> [w191 w231 w335 w341 w351 w355 w361 w373 w381 w387 w400 w413 w439 w452 w460 w464 w469 w478 w492 w508 w510 w518 w529 w534]
      tunnel: w176 -> [_ _ _ _ _ _ _ _ _ _ _ _ _ _ _ _ _ _ w493 _ w513 _ _ _]
      tunnel: w174 -> [_ _ _ _ _ _ _ _ _ _ _ _ _ _ _ _ _ _ w488 _ _ _ _ _]
      tunnel: w173 -> [_ _ _ _ _ _ _ _ _ _ _ _ _ _ _ _ _ _ w484 _ _ _ _ _]
      tunnel: w172 -> [w186 _ _ _ _ _ w359 _ _ _ _ _ _ _ _ _ _ _ _ _ _ _ _ _]
      tunnel: [w185 w230 w334 w340 w350 w356 w357 w367 w378 w386 w399 w412 w438 w451 w459 w463 w468 w477 w483 w506 w509 w514 w522 w535] -> w171
      tunnel: w170 -> [w185 w230 w334 w340 w350 w356 w357 _ _ w386 w399 w412 w438 w451 w459 w463 w468 w477 w483 w506 w509 w514 w522 w535]
      event Timeout {
        n94 = event-data() -> ()  [unwired: 1 in, 1 out]
        n95 = local read "Mode"() -> (w188:T6)
        n96 = call <vilib>:"NT Read String.vi"("Name"="/TestMode/TestName") -> ("String"=w197:string)  [unwired: 9 in, 1 out]
        n97 = case shown="\"Custom\", Default" "Dashboard Tab" {
          tunnel: w194 -> [_ w208 _ _]
          tunnel: "/TestMode/Automatic/" ("Name Pattern") -> [_ w207 _ _]
          tunnel: T25 [{"Operation"=enum."Clear", "Color Box"=14013909}, {"Operation"=enum."Clear", "Color Box"=14013909}, {"Operation"=enum."Clear", "Color Box"=14013909}, {"Operation"=enum."Clear", "Color Box"=14013909}, {"Operation"=enum."Update", "Color Box"=14013909}, {"Operation"=enum."Update", "Color Box"=16777215}, {"Operation"=enum."Clear", "Color Box"=14013909}, {"Operation"=enum."Clear", "Color Box"=14013909}, {"Operation"=enum."Clear", "Color Box"=14013909}] -> [_ w200 _ w217]
          tunnel: w188 -> [_ w199 _ w216]
          tunnel: u32[] [15790320, 15790320, 15790320, 15790320, 16777215, 16777215, 15790320, 15790320, 15790320] -> [_ _ _ w222]
          tunnel: w186 -> [_ _ _ w210]
          frame "Custom", Default {
          }
          frame "Test" {
            w206 = -2 ("Active Item:Row Number")
            n98 = Index Array(array=w200, index=w199) -> (element=w201:T29)
            n99 = Unbundle(w201) -> ("Operation"=w202:enum16{"Update", "Clear"}, "Color Box"=w203:u32)
            n100 = call <vilib>:"NT Read and Format Entries as Tree.vi"("Operation"=w202, "Name Pattern"=w207, "Tree Refnum"=w208) -> ()  [unwired: 7 in, 2 out]
            n101 = property on="Test Tree" class="Tree (strict)"("Active Item Row Number"=w206, "ActiveColNum"=w206, "CellBG"=w203, "Active Item Row Number"=-1 ("Active Item:Row Number"), "CellBG"=u32 5789784 ("Color Box")) -> ()  [unwired: 2 in, 2 out]
          }
          frame "Variables" {
            n102 = control-ref of="Tree"() -> (w209:refnum<vi>)
            n103 = call <vilib>:"NT Read and Format Entries as Tree.vi"("Tree Refnum"=w209) -> ()  [unwired: 9 in, 2 out]
          }
          frame "Commands" {
            w218 = u32 5789784 ("Color Box")
            w219 = T30 {"Row"=-1, "Column"=-2} ("Active Cell:Active Cell")
            w221 = T30 {"Row"=-2, "Column"=-2} ("Active Cell:Active Cell")
            n104 = Index Array(array=w222, index=w216) -> (element=w220:u32)
            n105 = Index Array(array=w217, index=w216) -> (element=w215:T29)
            n106 = Unbundle(w215) -> ("Operation"=w214:enum16{"Update", "Clear"})  [unwired: 1 out]
            n107 = local read "Command Selection"() -> (w213:i32)
            n108 = property on="Command Selection" class="MCListbox (strict)"("ActiveCell"=w221, "CellBG"=w220, "ActiveCell"=w219, "CellBG"=w218) -> ()  [unwired: 2 in, 2 out]
            n109 = call <vilib>:"WPI_DashboardUpdate RPC Info.vi"("Operation"=w214) -> ("update"=w212:bool, "commands"=w211:string[][])  [unwired: 9 in]
            n110 = property on="Command Selection" class="MCListbox (strict)"("ItemNames"=w211) -> ()  [unwired: 2 in, 2 out]
            n111 = property on="Command Params" class="Tbl (strict)"("Active Cell"=w221, "Cell BG Color"=w220, "Active Cell"=w219, "Cell BG Color"=w218) -> ()  [unwired: 2 in, 2 out]
            n112 = call <vilib>:"WPI_DashboardUpdate Command Params.vi"("Update"=w212, "NewVal"=w213, "Commands"=w211, "Param Tbl"=w210) -> ()  [unwired: 7 in, 1 out]
          }
        }
        n113 = case shown="\"\"" w197 {
          tunnel: "/TestMode/TestProgress" ("Name") -> [w224 _]
          tunnel: "/TestMode/TestProgressText" ("Name") -> [w223 _]
          frame Default {
            n114 = call <vilib>:"NT Read Number.vi"("Name"=w224) -> ("Numeric"=w225:dbl)  [unwired: 9 in, 1 out]
            n115 = call <vilib>:"NT Read String.vi"("Name"=w223) -> ("String"=w226:string)  [unwired: 9 in, 1 out]
            n116 = Bundle("Numeric"=w225, "String"=w226) -> (→"Progress":cluster{"Numeric":dbl, "String":string})  [unwired: 1 in]
          }
          frame "" {
            n117 = property on="Progress" class="Clust (strict)"("Visible"=FALSE) -> ()  [unwired: 2 in, 2 out]
            n118 = local write "Test Name"(u16 0) -> ()
          }
        }
        n119 = call <vilib>:"Connextion Info.vi"() -> ("Connected"=→"NT Connection":bool)  [unwired: 10 in, 1 out]
      }
      event "Test Tree": Value Change {
        # "Show appropriate\ncontrols"
        n120 = event-data() -> ("CtlRef"=w235:refnum<vi>, "NewVal"=w233:string)  [unwired: 1 in]
        n121 = call <vilib>:"WPI_UtilitiesGetTreeIOName.vi"("NewVal"=w233, "TreeControl in"=w235) -> ("I/O Name"=w236:string)  [unwired: 9 in]
        n122 = case shown="\"Analog Out\", \"Motor\", \"PWM\"" w236 {
          selector: w236 -> [_ w243 _ w265 w274 _]
          tunnel: w233 -> [_ _ w262 w264 _ w281]
          tunnel: w232 -> [_ _ _ _ _ w280]
          frame Default {
            w238 = FALSE ("Visible")
            w237 = FALSE ("Visible")
            n123 = property on="Motor" class="Clust (strict)"("Visible"=w237) -> ()  [unwired: 2 in, 2 out]
            n124 = property on="Test Ring" class="Ring (strict)"("Visible"=w237) -> ()  [unwired: 2 in, 2 out]
            n125 = property on="Rev/Fwd" class="Clust (strict)"("Visible"=w238) -> ()  [unwired: 2 in, 2 out]
            n126 = property on="On/Off" class="Bool (strict)"("Visible"=w238) -> ()  [unwired: 2 in, 2 out]
            n127 = property on="Test Slider" class="Slide (strict)"("Visible"=w238) -> ()  [unwired: 2 in, 2 out]
          }
          frame "Analog Out", "Motor", "PWM" {
            w244 = FALSE ("Visible")
            n128 = case shown="\"Analog Out\"" w243 {
              tunnel: [1.0 ("Value") -1.0 ("Value") 0.0 ("Value")] -> w242
              tunnel: [255.0 ("Value") 1.0 ("Value") 5.0 ("Value")] -> w241
              tunnel: [128.0 ("Value") 0.0 ("Value") 0.0 ("Value")] -> w240
              tunnel: [64.0 ("Value") 0.5 ("Value") 1.0 ("Value")] -> w239
              frame "PWM" {
              }
              frame "Motor", Default {
              }
              frame "Analog Out" {
              }
            }
            n129 = property on="Motor" class="Clust (strict)"("Visible"=TRUE) -> ()  [unwired: 2 in, 2 out]
            n130 = property on="Value" class="Slide (strict)"("Value"=w240, "Scale.Minimum"=w242, "Scale.Maximum"=w241, "Scale.Increment"=w239) -> ()  [unwired: 2 in, 2 out]
            n131 = property on="On/Off" class="Bool (strict)"("Visible"=w244) -> ()  [unwired: 2 in, 2 out]
            n132 = property on="Test Slider" class="Slide (strict)"("Visible"=w244) -> ()  [unwired: 2 in, 2 out]
            n133 = property on="Test Ring" class="Ring (strict)"("Visible"=w244) -> ()  [unwired: 2 in, 2 out]
            n134 = property on="Rev/Fwd" class="Clust (strict)"("Visible"=w244) -> ()  [unwired: 2 in, 2 out]
          }
          frame "Servo" {
            w260 = FALSE ("Visible")
            n135 = call <vilib>:"NT Read Number.vi"("Name"=w262) -> ("Numeric"=w261:dbl)  [unwired: 9 in, 1 out]
            n136 = property on="Test Slider" class="Slide (strict)"("Visible"=TRUE, "Scale.Maximum"=170.0 ("Scale.Range:Maximum")) -> ()  [unwired: 2 in, 2 out]
            n137 = local write "Test Slider"(w261) -> ()
            n138 = property on="Motor" class="Clust (strict)"("Visible"=w260) -> ()  [unwired: 2 in, 2 out]
            n139 = property on="Rev/Fwd" class="Clust (strict)"("Visible"=w260) -> ()  [unwired: 2 in, 2 out]
            n140 = property on="On/Off" class="Bool (strict)"("Visible"=w260) -> ()  [unwired: 2 in, 2 out]
            n141 = property on="Test Ring" class="Ring (strict)"("Visible"=w260) -> ()  [unwired: 2 in, 2 out]
          }
          frame "Relay", "Solenoid" {
            w263 = FALSE ("Visible")
            n142 = property on="Motor" class="Clust (strict)"("Visible"=w263) -> ()  [unwired: 2 in, 2 out]
            n143 = property on="Test Slider" class="Slide (strict)"("Visible"=w263) -> ()  [unwired: 2 in, 2 out]
            n144 = Search and Replace String(input string=w264, search string="/Value  **", replace string="/Direction") -> (result string=w270:string)  [unwired: 5 in, 3 out]
            n145 = property on="Test Ring" class="Ring (strict)"("Visible"=w263) -> ()  [unwired: 2 in, 2 out]
            n146 = call <vilib>:"NT Read String.vi"("Name"=w270) -> ("String"=w268:string)  [unwired: 9 in, 1 out]
            n147 = Equal?(x="Both directions", y=w268) -> (x = y?=w266:bool)
            n148 = Not(x=w266) -> (.not. x?=w267:bool)
            n149 = property on="Rev/Fwd" class="Clust (strict)"("Visible"=w266) -> ()  [unwired: 2 in, 2 out]
            n150 = property on="On/Off" class="Bool (strict)"("Visible"=w267, "Caption.Text"=w265) -> ()  [unwired: 2 in, 2 out]
          }
          frame "Compressor", "Digital Out" {
            w273 = FALSE ("Visible")
            # "Get direction and finish"
            n151 = property on="Motor" class="Clust (strict)"("Visible"=w273) -> ()  [unwired: 2 in, 2 out]
            n152 = property on="Test Slider" class="Slide (strict)"("Visible"=w273) -> ()  [unwired: 2 in, 2 out]
            n153 = property on="Test Ring" class="Ring (strict)"("Visible"=w273) -> ()  [unwired: 2 in, 2 out]
            n154 = property on="On/Off" class="Bool (strict)"("Visible"=TRUE, "Caption.Text"=w274) -> ()  [unwired: 2 in, 2 out]
            n155 = property on="Rev/Fwd" class="Clust (strict)"("Visible"=FALSE) -> ()  [unwired: 2 in, 2 out]
          }
          frame "Camera" {
            n156 = call <vilib>:"Get Last Path Segment.vi"("String in"=w281) -> ("String out"=w282:string)  [unwired: 10 in]
            n157 = property on="On/Off" class="Bool (strict)"("Visible"=FALSE) -> ()  [unwired: 2 in, 2 out]
            n158 = property on="Motor" class="Clust (strict)"("Visible"=FALSE) -> ()  [unwired: 2 in, 2 out]
            n159 = property on="Rev/Fwd" class="Clust (strict)"("Visible"=FALSE) -> ()  [unwired: 2 in, 2 out]
            n160 = case shown="\"White Balance  **\"" w282 {
              tunnel: w281 -> [w288 w297 w306 w315 w324 _ w330]
              tunnel: w280 -> [w286 w294 w303 w312 w321 _ _]
              frame "Size  **" {
                n161 = Index Array(array=w286) -> (element=w285:cluster{string[]})  [unwired: 1 in]
                n162 = call <vilib>:"NT Read String.vi"("Name"=w288) -> ("String"=w287:string)  [unwired: 9 in, 1 out]
                n163 = Unbundle(w285) -> (w283:string[])
                n164 = Match First String(2:w283, 3:w287) -> (0:w284:i32)  [unwired: 1 out]
                n165 = property on="Test Ring" class="Ring (strict)"("Value"=w284, "Strings []"=w283) -> ()  [unwired: 2 in, 2 out]
                n166 = property on="Test Ring" class="Ring (strict)"("Visible"=TRUE) -> ()  [unwired: 2 in, 2 out]
                n167 = property on="Test Slider" class="Slide (strict)"("Visible"=FALSE) -> ()  [unwired: 2 in, 2 out]
              }
              frame "White Balance  **" {
                n168 = Index Array(array=w294, index=1) -> (element=w295:cluster{string[]})
                n169 = call <vilib>:"NT Read String.vi"("Name"=w297) -> ("String"=w296:string)  [unwired: 9 in, 1 out]
                n170 = Unbundle(w295) -> (w292:string[])
                n171 = Match First String(2:w292, 3:w296) -> (0:w291:i32)  [unwired: 1 out]
                n172 = property on="Test Ring" class="Ring (strict)"("Value"=w291, "Strings []"=w292) -> ()  [unwired: 2 in, 2 out]
                n173 = property on="Test Ring" class="Ring (strict)"("Visible"=TRUE) -> ()  [unwired: 2 in, 2 out]
                n174 = property on="Test Slider" class="Slide (strict)"("Visible"=FALSE) -> ()  [unwired: 2 in, 2 out]
              }
              frame "Exposure  **" {
                n175 = Index Array(array=w303, index=2) -> (element=w304:cluster{string[]})
                n176 = call <vilib>:"NT Read String.vi"("Name"=w306) -> ("String"=w305:string)  [unwired: 9 in, 1 out]
                n177 = Unbundle(w304) -> (w300:string[])
                n178 = Match First String(2:w300, 3:w305) -> (0:w301:i32)  [unwired: 1 out]
                n179 = property on="Test Ring" class="Ring (strict)"("Value"=w301, "Strings []"=w300) -> ()  [unwired: 2 in, 2 out]
                n180 = property on="Test Ring" class="Ring (strict)"("Visible"=TRUE) -> ()  [unwired: 2 in, 2 out]
                n181 = property on="Test Slider" class="Slide (strict)"("Visible"=FALSE) -> ()  [unwired: 2 in, 2 out]
              }
              frame "Exposure Priority  **" {
                n182 = Index Array(array=w312, index=3) -> (element=w313:cluster{string[]})
                n183 = call <vilib>:"NT Read String.vi"("Name"=w315) -> ("String"=w314:string)  [unwired: 9 in, 1 out]
                n184 = Unbundle(w313) -> (w309:string[])
                n185 = Match First String(2:w309, 3:w314) -> (0:w310:i32)  [unwired: 1 out]
                n186 = property on="Test Ring" class="Ring (strict)"("Value"=w310, "Strings []"=w309) -> ()  [unwired: 2 in, 2 out]
                n187 = property on="Test Ring" class="Ring (strict)"("Visible"=TRUE) -> ()  [unwired: 2 in, 2 out]
                n188 = property on="Test Slider" class="Slide (strict)"("Visible"=FALSE) -> ()  [unwired: 2 in, 2 out]
              }
              frame "Color Enable  **" {
                n189 = Index Array(array=w321, index=4) -> (element=w322:cluster{string[]})
                n190 = call <vilib>:"NT Read String.vi"("Name"=w324) -> ("String"=w323:string)  [unwired: 9 in, 1 out]
                n191 = Unbundle(w322) -> (w318:string[])
                n192 = Match First String(2:w318, 3:w323) -> (0:w319:i32)  [unwired: 1 out]
                n193 = property on="Test Ring" class="Ring (strict)"("Value"=w319, "Strings []"=w318) -> ()  [unwired: 2 in, 2 out]
                n194 = property on="Test Ring" class="Ring (strict)"("Visible"=TRUE) -> ()  [unwired: 2 in, 2 out]
                n195 = property on="Test Slider" class="Slide (strict)"("Visible"=FALSE) -> ()  [unwired: 2 in, 2 out]
              }
              frame Default {
                n196 = property on="Test Ring" class="Ring (strict)"("Visible"=FALSE) -> ()  [unwired: 2 in, 2 out]
                n197 = property on="Test Slider" class="Slide (strict)"("Visible"=FALSE) -> ()  [unwired: 2 in, 2 out]
              }
              frame "Brightness  **", "Color Level  **", "Compression  **", "FPS  **", "Sharpness  **" {
                n198 = call <vilib>:"NT Read Number.vi"("Name"=w330) -> ("Numeric"=w329:dbl)  [unwired: 9 in, 1 out]
                n199 = local write "Test Slider"(w329) -> ()
                n200 = property on="Test Slider" class="Slide (strict)"("Visible"=TRUE, "Scale.Maximum"=100.0 ("Scale.Range:Maximum")) -> ()  [unwired: 2 in, 2 out]
                n201 = property on="Test Ring" class="Ring (strict)"("Visible"=FALSE) -> ()  [unwired: 2 in, 2 out]
              }
            }
          }
        }
        n202 = property on="Progress" class="Clust (strict)"("Visible"=FALSE) -> ()  [unwired: 2 in, 2 out]
      }
      event "Test Name": Mouse Enter {
        # "Populate the ring with the list of tests"
        n203 = event-data() -> ()  [unwired: 1 in, 1 out]
        n204 = call <vilib>:"NT Read String Array.vi"("Name"="/TestMode/TestList") -> ("String Array"=w339:string[])  [unwired: 9 in, 1 out]
        n205 = Build Array (concatenate)("Select the test to run...", w339) -> (w338:string[])
        n206 = property on="Test Name" class="Ring (strict)"("Strings []"=w338) -> ()  [unwired: 2 in, 2 out]
      }
      event "Test Name": Value Change {
        w342 = FALSE ("Visible")
        # "Tell the robot the test name to run"
        n207 = event-data() -> ("NewVal"=w346:u16)  [unwired: 1 in]
        n208 = property on="Test Name" class="Ring (strict)"() -> ("Strings []"=w347:string[])  [unwired: 2 in, 2 out]
        n209 = local write "Progress"(T8 {"Test Progress"=0, "Test Progress Text"=""} ("Progress")) -> ()
        n210 = Index Array(array=w347, index=w346) -> (element=w345:string)
        n211 = call <vilib>:"NT Write String.vi"("String"=w345, "Name"="/TestMode/TestName") -> ()  [unwired: 9 in, 1 out]
        n212 = property on="Progress" class="Clust (strict)"("Visible"=TRUE) -> ()  [unwired: 2 in, 2 out]
        n213 = property on="Motor" class="Clust (strict)"("Visible"=w342) -> ()  [unwired: 2 in, 2 out]
        n214 = property on="Test Slider" class="Slide (strict)"("Visible"=w342) -> ()  [unwired: 2 in, 2 out]
        n215 = property on="On/Off" class="Bool (strict)"("Visible"=w342) -> ()  [unwired: 2 in, 2 out]
        n216 = property on="Rev/Fwd" class="Clust (strict)"("Visible"=w342) -> ()  [unwired: 2 in, 2 out]
        n217 = property on="Test Ring" class="Ring (strict)"("Visible"=w342) -> ()  [unwired: 2 in, 2 out]
      }
      event "Select Auto": Mouse Enter {
        # "Populate the combo box with the list of autonomous options"
        n218 = event-data() -> ()  [unwired: 1 in, 1 out]
        n219 = call <vilib>:"NT Read String Array.vi"("Name"="Auto List") -> ("String Array"=w349:string[])  [unwired: 9 in, 1 out]
        n220 = property on="Select Auto" class="CmbBox"("Strings[]"=w349) -> ()  [unwired: 2 in, 2 out]
      }
      event "Select Auto": Value Change {
        # "User modified the Auto Selection. Write to NT variable so robot knows."
        n221 = event-data() -> ("NewVal"=w353:string)  [unwired: 1 in]
        n222 = call <vilib>:"NT Write String.vi"("String"=w353, "Name"="Auto Selector") -> ()  [unwired: 9 in, 1 out]
      }
      event "Command Selection": Value Change {
        # "Get the params and show in table"
        n223 = event-data() -> ("NewVal"=w360:i32)  [unwired: 1 in]
        n224 = property on="Command Selection" class="MCListbox (strict)"() -> ("ItemNames"=w358:string[][])  [unwired: 2 in, 2 out]
        n225 = call <vilib>:"WPI_DashboardUpdate Command Params.vi"("NewVal"=w360, "Commands"=w358, "Param Tbl"=w359) -> ()  [unwired: 8 in, 1 out]
      }
      event "Execute Command": Value Change {
        # "Started one, Unique ID holds\nresponse"
        n226 = event-data() -> ()  [unwired: 1 in, 1 out]
        n227 = property on="Command Selection" class="MCListbox (strict)"() -> ("ItemNames"=w372:string[][])  [unwired: 2 in, 2 out]
        n228 = Index Array(array=w372, index (row)="Command Selection", index (col)=0) -> (element=w370:string)
        n229 = call <vilib>:"Invoke Commands.vi"("Command Params"="Command Params", "Function Name"=w370) -> ("Params"=w366:u8, "Started"=w365:bool)  [unwired: 7 in, 1 out]
        n230 = Array Subset(array="Command Params", length (row)=w366) -> (w367:string[][])  [unwired: 3 in]
        n231 = Select(t="Executing" ("Cmd Status"), s=w365, f="" ("Cmd Status")) -> (s? t:f=→"Cmd Status":string)
      }
      event "Command Selection": Double Click {
        n232 = event-data() -> ("Row"=w382:i32)  [unwired: 1 in]
        n233 = property on="Command Selection" class="MCListbox (strict)"() -> ("ItemNames"=w385:string[][])  [unwired: 2 in, 2 out]
        n234 = local read "Command Params"() -> (w380:string[][])
        n235 = Index Array(array=w385, index (row)=w382, index (col)=0) -> (element=w383:string)
        n236 = call <vilib>:"Invoke Commands.vi"("Command Params"=w380, "Function Name"=w383) -> ("Params"=w379:u8, "Started"=w374:bool)  [unwired: 7 in, 1 out]
        n237 = Array Subset(array=w380, length (row)=w379) -> (w378:string[][])  [unwired: 3 in]
        n238 = Select(t="Executing" ("Cmd Status"), s=w374, f="" ("Cmd Status")) -> (s? t:f=w375:string)
        n239 = local write "Cmd Status"(w375) -> ()
      }
      event "CheckList": Double Click {
        # "Shift clears all"
        # "Update symbols on the listbox"
        n240 = event-data() -> ("PlatMods.Shift"=w388:bool, "Row"=w390:i32)  [unwired: 1 in]
        n241 = case shown="True" w388 {
          tunnel: w390 -> [w394 _]
          tunnel: 1 -> [w393 _]
          frame False {
            n242 = property on="CheckList" class="LstBox (strict)"() -> ("Item Symbols"=w392:i32[])  [unwired: 2 in, 2 out]
            n243 = Replace Array Subset(array=w392, new element=w393, index=w394) -> (w391:i32[])
            n244 = property on="CheckList" class="LstBox (strict)"("Item Symbols"=w391) -> ()  [unwired: 2 in, 2 out]
          }
          frame True {
            w395 = 0 ("Top Row")
            n245 = property on="CheckList" class="LstBox (strict)"() -> ("Number of Rows"=w397:u32)  [unwired: 2 in, 2 out]
            n246 = Initialize Array(0, w397) -> (w396:i32[])
            n247 = property on="CheckList" class="LstBox (strict)"("Top Row"=w395, "Value"=w395, "Item Symbols"=w396) -> ()  [unwired: 2 in, 2 out]
          }
        }
      }
      event "CheckList": Key Down {
        # "Update symbols on the listbox\nLeft and right keys check and uncheck"
        n248 = event-data() -> ("VKey"=w402:T26)  [unwired: 1 in]
        n249 = case shown="\"Left\", \"Right\"" w402 {
          selector: w402 -> [w407 _]
          tunnel: eventvkey."Left" ("VKey") -> [w405 _]
          frame "Left", "Right" {
            n250 = Equal?(x=w405, y=w407) -> (x = y?=w406:bool)
            n251 = Select(t=0, s=w406, f=1) -> (s? t:f=w408:i32)
            n252 = property on="CheckList" class="LstBox (strict)"() -> ("Item Symbols"=w411:i32[])  [unwired: 2 in, 2 out]
            n253 = Replace Array Subset(array=w411, new element=w408, index="CheckList") -> (w410:i32[])
            n254 = property on="CheckList" class="LstBox (strict)"("Item Symbols"=w410) -> ()  [unwired: 2 in, 2 out]
          }
          frame Default {
          }
        }
      }
      event "DB Camera Config": Value Change {
        # "Show or hide the cluster of controls, store in ini file"
        n255 = event-data() -> ("NewVal"=w416:bool)  [unwired: 1 in]
        n256 = case shown="False" w416 {
          tunnel: w415 -> [w425 _]
          tunnel: [w418 w436] -> w414
          tunnel: w413 -> [w417 w436]
          frame False {
            w432 = "Camera"
            w435 = FALSE ("Visible")
            n257 = local read "Camera Settings"() -> (w424:T2)
            n258 = Index Array(array=w425) -> (element=w428:cluster{string[]})  [unwired: 1 in]
            n259 = Unbundle(w424) -> ("Frame Rate"=w423:i32, "Compression"=w422:i32, "Size"=w426:u16)
            n260 = Unbundle(w428) -> (w427:string[])
            n261 = Index Array(array=w427, index=w426) -> (element=w421:string)
            n262 = call-poly <vilib>:"Write Key.vi"("section"=w432, "value"=w421, "key"="Size", "refnum"=w417) -> ("refnum out"=w434:T24)  [unwired: 2 in, 5 out]
            n263 = call-poly <vilib>:"Write Key.vi"("section"=w432, "value"=w423, "key"="FrameRate", "refnum"=w434) -> ("refnum out"=w433:T24)  [unwired: 1 in, 6 out]
            n264 = property on="Camera Settings" class="Clust (strict)"("Visible"=w435) -> ()  [unwired: 2 in, 2 out]
            n265 = local write "DB Camera Config"(w435) -> ()
            n266 = call-poly <vilib>:"Write Key.vi"("section"=w432, "value"=w422, "key"="Compression", "refnum"=w433) -> ("refnum out"=w419:T24)  [unwired: 1 in, 6 out]
            n267 = call <vilib>:"Close Config Data.vi"("refnum"=w419) -> ("file path"=w420:path)  [unwired: 2 in, 8 out]
            n268 = call <vilib>:"Open Config Data.vi"("configuration file path"=w420) -> ("refnum"=w418:T24)  [unwired: 8 in, 2 out]
          }
          frame True {
            n269 = property on="Camera Settings" class="Clust (strict)"("Visible"=TRUE) -> ()  [unwired: 2 in, 2 out]
          }
        }
      }
      event "Camera Settings": Value Change {
        # "Update summary string when any elements of DB camera change"
        n270 = event-data() -> ("NewVal"=w450:T2)  [unwired: 1 in]
        n271 = Index Array(array=w446) -> (element=w445:cluster{string[]})  [unwired: 1 in]
        n272 = Unbundle(w450) -> ("Frame Rate"=w441:i32, "Compression"=w440:i32, "Size"=w443:u16)
        n273 = Unbundle(w445) -> (w444:string[])
        n274 = Index Array(array=w444, index=w443) -> (element=w442:string)
        n275 = Format Into String(format string="%s   %dfps   %d%%", w442, w441, w440) -> (resulting string=w447:string)  [unwired: 2 in, 1 out]
        n276 = Build Array(w447) -> (w448:string[])
        n277 = property on="DB Camera Config" class="Bool (strict)"("Strings [4]"=w448) -> ()  [unwired: 2 in, 2 out]
      }
      event "Motor.Enable": Value Change {
        # "When the test mode otor enable helper is set, update that\ntree row item's value"
        n278 = event-data() -> ("NewVal"=w457:bool)  [unwired: 1 in]
        n279 = Unbundle("Motor") -> ("Value"=w456:dbl)  [unwired: 1 out]
        n280 = Select(t=w456, s=w457, f=0.0) -> (s? t:f=w454:dbl)
        n281 = call <vilib>:"NT Write Number.vi"("Numeric"=w454, "Name"=w453) -> ()  [unwired: 9 in, 1 out]
      }
      event "Test Slider": Value Change {
        # "When the test mode slider helper is set, update that\ntree row item's value"
        n282 = event-data() -> ("NewVal"=w461:dbl)  [unwired: 1 in]
        n283 = call <vilib>:"NT Write Number.vi"("Numeric"=w461, "Name"=w462) -> ()  [unwired: 9 in, 1 out]
      }
      event "On/Off": Value Change {
        # "When the test mode on/off helper value is set, update that\ntree row item's value"
        n284 = event-data() -> ("NewVal"=w467:bool)  [unwired: 1 in]
        n285 = Boolean To (0,1)(Boolean=w467) -> (0, 1=w466:i16)
        n286 = call <vilib>:"NT Write Number.vi"("Numeric"=w466, "Name"=w465) -> ()  [unwired: 9 in, 1 out]
      }
      event "Rev/Fwd": Value Change {
        # "When the test mode helper value for relays is set, update that\ntree row item's value"
        n287 = event-data() -> ("NewVal.Forward"=w476:bool, "NewVal.Reverse"=w475:bool)  [unwired: 1 in]
        n288 = Boolean To (0,1)(Boolean=w476) -> (0, 1=w472:i16)
        n289 = Boolean To (0,1)(Boolean=w475) -> (0, 1=w474:i16)
        n290 = Negate(x=w474) -> (-x=w473:i16)
        n291 = Add(x=w472, y=w473) -> (x+y=w471:i16)
        n292 = call <vilib>:"NT Write Number.vi"("Numeric"=w471, "Name"=w470) -> ()  [unwired: 9 in, 1 out]
      }
      event "Test Ring": Value Change {
        # "When a test mode helper value is selected from the ring,\nset the tree item's variable to the string value"
        n293 = event-data() -> ("NewVal"=w481:u16)  [unwired: 1 in]
        n294 = property on="Test Ring" class="Ring (strict)"() -> ("Strings []"=w482:string[])  [unwired: 2 in, 2 out]
        n295 = Index Array(array=w482, index=w481) -> (element=w480:string)
        n296 = call <vilib>:"NT Write String.vi"("String"=w480, "Name"=w479) -> ()  [unwired: 9 in, 1 out]
      }
      event "Rec Mode": Value Change {
        # "Update globals for recording mode and path to read log from.\nClear when logging and let NetworkTables set path for vision to\nuse."
        n297 = event-data() -> ("NewVal"=w494:enum32{"Stop", "Record", "Playback"})  [unwired: 1 in]
        n298 = global write "WPI_DashboardLogging Global.vi" "Logging Filename"(path "") -> ()
        n299 = global write "WPI_DashboardLogging Global.vi" "Recording"(w494) -> ()
        n300 = case shown="\"Playback\"" w494 {
          tunnel: w493 -> [_ w496 w505]
          tunnel: [_ _ w504] -> w490
          tunnel: [_ _ w503] -> _
          tunnel: w488 -> [_ _ w501]
          tunnel: cluster{i32, i32} {-250, 170} -> [_ _ w500]
          tunnel: [_ _ T27 {"Image Size"=TRUE, "Image Type"=TRUE, "Pixel Value"=TRUE, "ROI Information"=TRUE, "Zoom Factor"=FALSE} ("Image Information Shown:All Elements")] -> w486
          tunnel: [_ _ TRUE ("Zoom Factor")] -> w485
          tunnel: w484 -> [_ _ w497]
          frame Default {
          }
          frame "Stop", "Record" {
            # "Place Window too"
            n301 = invoke class="VI" method="FP.Close"(reference=w496) -> (reference out=w495:refnum<vi>)  [unwired: 2 in, 2 out]
            n302 = invoke class="VI" method="Abort VI"(reference=w495) -> ()  [unwired: 2 in, 3 out]
          }
          frame "Playback" {
            n303 = call "Open Playback Panel.vi"("Offset"=w500, "DB VI Ref"=w501, "Playback in"=w505) -> ("Playback out"=w502:refnum<vi>)  [unwired: 8 in]
            n304 = register-events(w502, w497) -> (reference out=w504:refnum<event-registration>, error out=w503:errorcluster)  [unwired: 2 in]
          }
        }
        n305 = property on="Camera Image" class="ImageControl"("Image Information Shown"=w486, "Image Information Visible"=w485) -> ()  [unwired: 2 in, 2 out]
        n306 = call <vilib>:"WPI_DashboardNT Log FieldName Cache.vi"("Operation"=enum16{"Lookup/Add", "Index", "Clear"}."Clear") -> ()  [unwired: 8 in, 3 out]
      }
      event Panel Close {
        w507 = enum32{"Stop", "Record", "Playback"}."Stop" ("Rec Mode")
        # "Playback window has been closed, abort"
        n307 = event-data() -> ()  [unwired: 1 in, 4 out]
        n308 = local write "Rec Mode"(w507) -> ()
        n309 = global write "WPI_DashboardLogging Global.vi" "Recording"(w507) -> ()
      }
      event Panel Close {
        # "Abort playback window and ourself"
        n310 = event-data() -> ()  [unwired: 1 in, 4 out]
        n311 = invoke class="VI" method="FP.Close"(reference=w513) -> (reference out=w512:refnum<vi>)  [unwired: 2 in, 2 out]
        n312 = invoke class="VI" method="Abort VI"(reference=w512) -> (error out=w511:errorcluster)  [unwired: 2 in, 2 out]
        n313 = invoke class="VI" method="Abort VI"(error in=w511) -> ()  [unwired: 2 in, 3 out]
      }
      event User Event {
        n314 = event-data() -> ("IDs"=w521:cluster{"RPC field ID":u16, "Unique ID":u16}, "String"=w520:string)  [unwired: 1 in]
        n315 = Bundle("IDs"=w521, "String"=w520) -> (w519:T12)  [unwired: 1 in]
        n316 = call <vilib>:"Retrieve RPC Response.vi"("RPC Response"=w519) -> ("Output"=w516:string[][])  [unwired: 10 in]
        n317 = Build Array (concatenate)(w514, w516) -> (w515:string[][])
        n318 = local write "Command Params"(w515) -> ()
        n319 = local write "Cmd Status"("" ("Cmd Status")) -> ()
      }
      event "Vision": Value Change {
        # "Enable/Disable Compression slider.\nHW USB is hard-coded into the camera"
        n320 = event-data() -> ("NewVal"=w528:u16)  [unwired: 1 in]
        n321 = Equal?(x=w528, y=u32 2 ("milliseconds to wait")) -> (x = y?=w526:bool)
        n322 = Select(t=T28."Disabled and Grayed Out" ("Disabled"), s=w526, f=T28."Enabled" ("Disabled")) -> (s? t:f=w523:T28)
        n323 = property on="Compression" class="Slide (strict)"("DisabledEnum"=w523) -> ()  [unwired: 2 in, 2 out]
      }
      event "Tree": Double Click {
        n324 = event-data() -> ("PlatMods"=w533:T31, "Tag"=w532:string)  [unwired: 1 in]
        n325 = Unbundle(w533) -> ("Shift"=w531:bool)  [unwired: 4 out]
        n326 = Not(x=w531) -> (.not. x?=w530:bool)
        n327 = call <vilib>:"NT Update Persistence.vi"("Persistence"=w530, "Name"=w532) -> ()  [unwired: 9 in, 1 out]
      }
    }
  }
  n328 = while {
    tunnel: w49 -> [w537]
    i -> [w540]
    stop <- FALSE stop-if-true
    n329 = Wait (ms)(milliseconds to wait=u32 100) -> ()  [unwired: 1 out]
    n330 = case shown="\"Stop\", Default" "Rec Mode" {
      tunnel: w540 -> [_ _ w555]
      tunnel: [u32 2829099 ("Base Color") u32 11141120 ("Target Color") w544] -> w536
      frame "Stop", Default {
        # "Reset the color, extra updates don't cost much"
      }
      frame "Record" {
      }
      frame "Playback" {
        # "Playback"
        n331 = Quotient & Remainder(x=w555, y=u32 50 ("milliseconds to wait")) -> (x-y*floor(x/y)=w551:u32)  [unwired: 1 out]
        n332 = Divide(x=w551, y=u32 50 ("milliseconds to wait")) -> (x/y=w548:dbl)
        n333 = Multiply(x=6.283185307179586, y=w548) -> (x*y=w553:dbl)
        n334 = Sine(x=w553) -> (sin(x)=w552:dbl)
        n335 = Absolute Value(x=w552) -> (abs(x)=w545:dbl)
        n336 = call "Interpolate RGB Color.vi"("Proportion"=w545, "Target Color"=u32 30976, "Base Color"=u32 2829099) -> ("Result Color"=w544:u32)  [unwired: 8 in]
      }
    }
    n337 = property class="Pane"(reference=w537, "PaneColor"=w536) -> ()  [unwired: 1 in, 2 out]
  }
  n338 = local write "Dashboard Tab"(T13."Drive" ("Dashboard Tab")) -> ()
  n339 = property on="On/Off" class="Bool (strict)"("Visible"=w17) -> ()  [unwired: 2 in, 2 out]
  n340 = property on="Motor" class="Clust (strict)"("Visible"=w17) -> ()  [unwired: 2 in, 2 out]
  n341 = property on="Progress" class="Clust (strict)"("Visible"=w17) -> ()  [unwired: 2 in, 2 out]
  n342 = property on="Test Ring" class="Ring (strict)"("Visible"=w17) -> ()  [unwired: 2 in, 2 out]
  n343 = property on="Rev/Fwd" class="Clust (strict)"("Visible"=w17) -> ()  [unwired: 2 in, 2 out]
  n344 = property on="Camera Settings" class="Clust (strict)"("Visible"=w17) -> ()  [unwired: 2 in, 2 out]
  n345 = local write "DB Camera Config"(w17) -> ()
  n346 = while {
    tunnel: u16 1741 ("timeout ms (25000)") -> [w557]
    stop <- FALSE stop-if-true
    n347 = TCP Create Listener(10:w557) -> (0:w556:errorcluster, 3:w558:refnum<k5>)  [unwired: 4 in, 1 out]
    n348 = case shown="No Error" w556 {
      selector: w556 -> [w560 _]
      tunnel: w558 -> [w561 _]
      frame No Error {
        n349 = while {
          tunnel: w561 -> [w564]
          tunnel: w560 -> [w563]
          stop <- FALSE stop-if-true
          n350 = TCP Wait On Listener(8:w563, 11:w564) -> (0:w565:errorcluster, 4:w566:refnum<k5>)  [unwired: 2 in, 3 out]
          n351 = local write "TCP"(w566) -> ()
          n352 = case shown="No Error" w565 {
            frame No Error {
            }
            frame Error {
              n353 = Wait (ms)(milliseconds to wait=u32 1000) -> ()  [unwired: 1 out]
            }
          }
        }
      }
      frame Error {
        n354 = Wait (ms)(milliseconds to wait=u32 1000) -> ()  [unwired: 1 out]
      }
    }
  }
  n355 = local write "Command Params"(string[][] [] ("Command Params")) -> ()
  n356 = global write "WPI_DashboardLogging Global.vi" "Recording"(w43) -> ()
  n357 = local write "Rec Mode"(w43) -> ()
  n358 = local write "Command Selection"(u16 0 ("milliseconds to wait")) -> ()
